vi "Make hexadecimal command for Sutter manipulator.vi"(6 "Zcommand (microns)":dbl format="%.4f", 8 "Ycommand (microns)":dbl format="%.4f", 9 "Xcommand (microns)":dbl format="%.4f", 10 "Manipulator":i32(ring) items=["1", "2", "3", "4"], 11 "Command":u16(ring) items=["Change manipulator", "Get current position", "Go to position", "Home", "Work", "Center", "Interrupt move", "Off"]) -> (3 "Hexadecimal command string":string)   [LabVIEW 2010]
panel:
  out "Zcommand (microns)":dbl format="%.4f"
  # "Set to hex display"
  # "http://www.sutter.com/software/usb.doc"
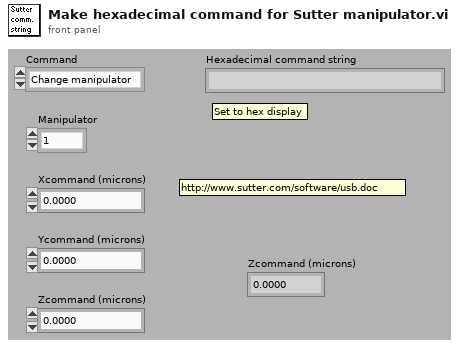
[diagram p1: front panel]
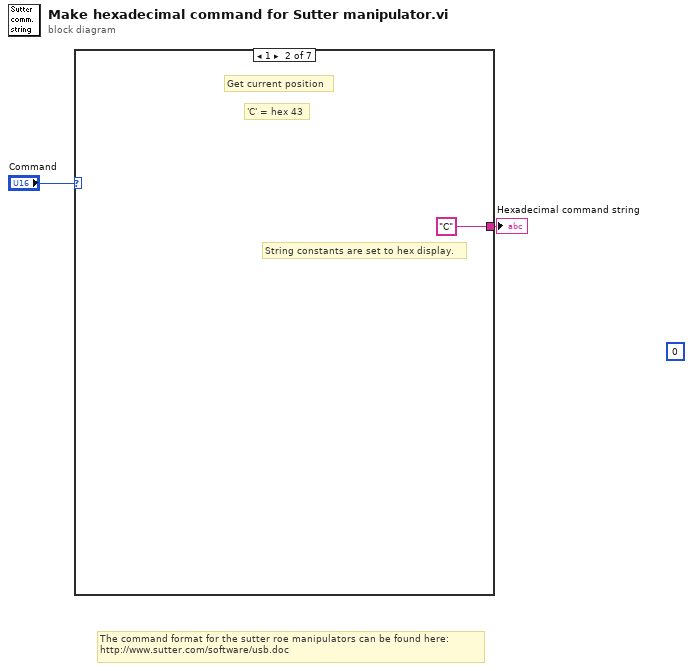
[diagram p0: block diagram]
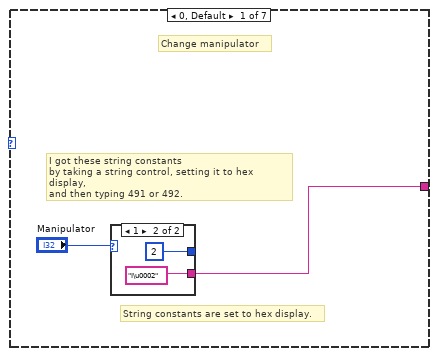
[diagram p2: hidden frame]
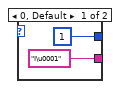
[diagram p3: hidden frame]
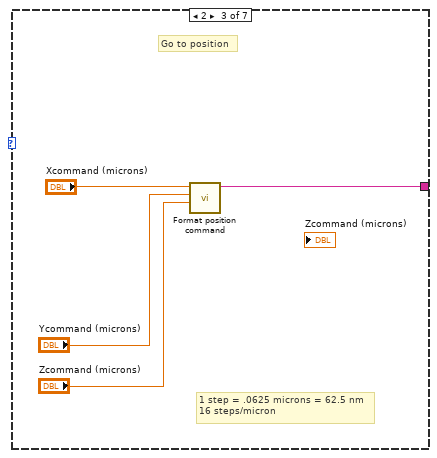
[diagram p4: hidden frame]
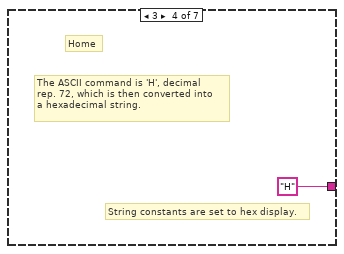
[diagram p5: hidden frame]
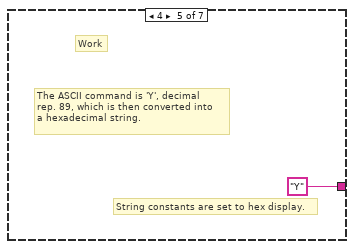
[diagram p6: hidden frame]
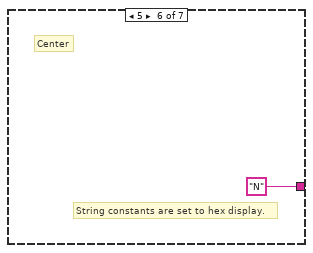
[diagram p7: hidden frame]
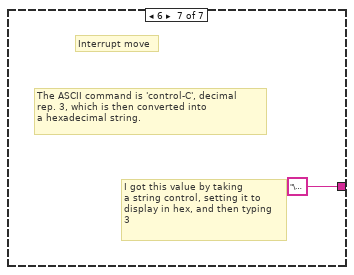
[diagram p8: hidden frame]
diagram:
  (unwired) 0
  # "The command format for the sutter roe manipulators can be found here:\nhttp://www.sutter.com/software/usb.doc"
  n1 = case shown="1" "Command" {
    tunnel: [w3 "C" w10 "H" "Y" "N" "\u0003"] -> w1
    frame 0, Default {
      # "String constants are set to hex display."
      # "I got these string constants\nby taking a string control, setting it to hex display,\nand then typing 491 or 492."
      # "Change manipulator"
      n2 = case shown="1" "Manipulator" {
        tunnel: [1 2] -> _
        tunnel: ["I\u0001" ("string") "I\u0002" ("string")] -> w3
        frame 0, Default {
        }
        frame 1 {
        }
      }
    }
    frame 1 {
      # "'C' = hex 43"
      # "String constants are set to hex display."
      # "Get current position"
    }
    frame 2 {
      # "1 step = .0625 microns = 62.5 nm\n16 steps/micron"
      # "Go to position"
      n3 = call "Format position command.vi"("Zcommand (steps)"="Zcommand (microns)", "Ycommand (steps)"="Ycommand (microns)", "Xcommand (steps)"="Xcommand (microns)") -> ("concatenated string"=w10:string)  [unwired: 8 out]
    }
    frame 3 {
      # "String constants are set to hex display."
      # "The ASCII command is 'H', decimal\nrep. 72, which is then converted into\na hexadecimal string."
      # "Home"
    }
    frame 4 {
      # "String constants are set to hex display."
      # "The ASCII command is 'Y', decimal\nrep. 89, which is then converted into\na hexadecimal string."
      # "Work"
    }
    frame 5 {
      # "String constants are set to hex display."
      # "Center"
    }
    frame 6 {
      # "I got this value by taking\na string control, setting it to\ndisplay in hex, and then typing\n3"
      # "The ASCII command is 'control-C', decimal\nrep. 3, which is then converted into\na hexadecimal string."
      # "Interrupt move"
    }
  }
  "Hexadecimal command string" <- w1
